vi "Experiment header-Save_Load STATS for Z-stack26_01_18.vi"(8 "error in (no error)":errorcluster, 10 "Function":enum16{"Write", "Read"}(ring), 11 "Experiment folder path":path) -> (0 "error out":errorcluster)   [LabVIEW 2017]
uses:
  Global Variables/General Globals.vi
  <vilib>/Utility/config.llb/Write Key (Double).vi
  <vilib>/Utility/config.llb/NI_LVConfig.lvlib
  <vilib>/Utility/config.llb/Read Key (Double).vi
panel:
  out "Z-stack duration (sec)":dbl
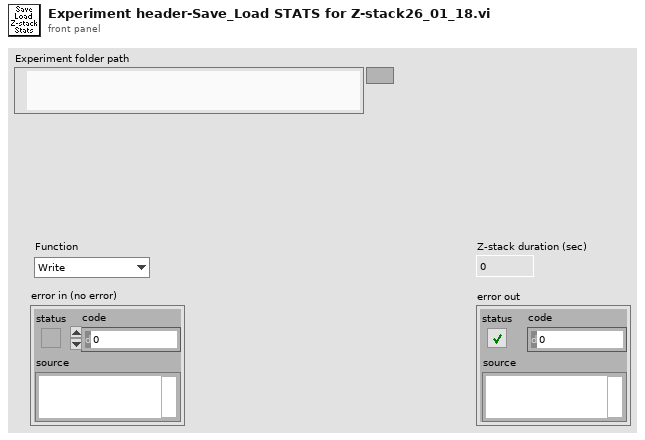
[diagram p1: front panel]
types:
  T1 = typedef "Fixed strings.ctl" = cluster{"ROI file name":string, "Normalised ROI file name":string, "Zplane Pockels values file name":string, "Functional data folder name":string, "Experiment Header file name":string, "Z-stack images folder name":string, "Groups setup rel. path":string, "Groups text file rel. path":string, "TDMS files folder name (F.img)":string, "TDMS files folder name (V.acq)":string, "TDMS files folder name (Pl.acq)":string, "Cycle rel times sequence file":string, "Dynamically called VIs folder name":string, "Time Series folder base name":string}
  T2 = typedef "NI_LVConfig.lvlib/Config Data RefNum.ctl" = refnum<k1>
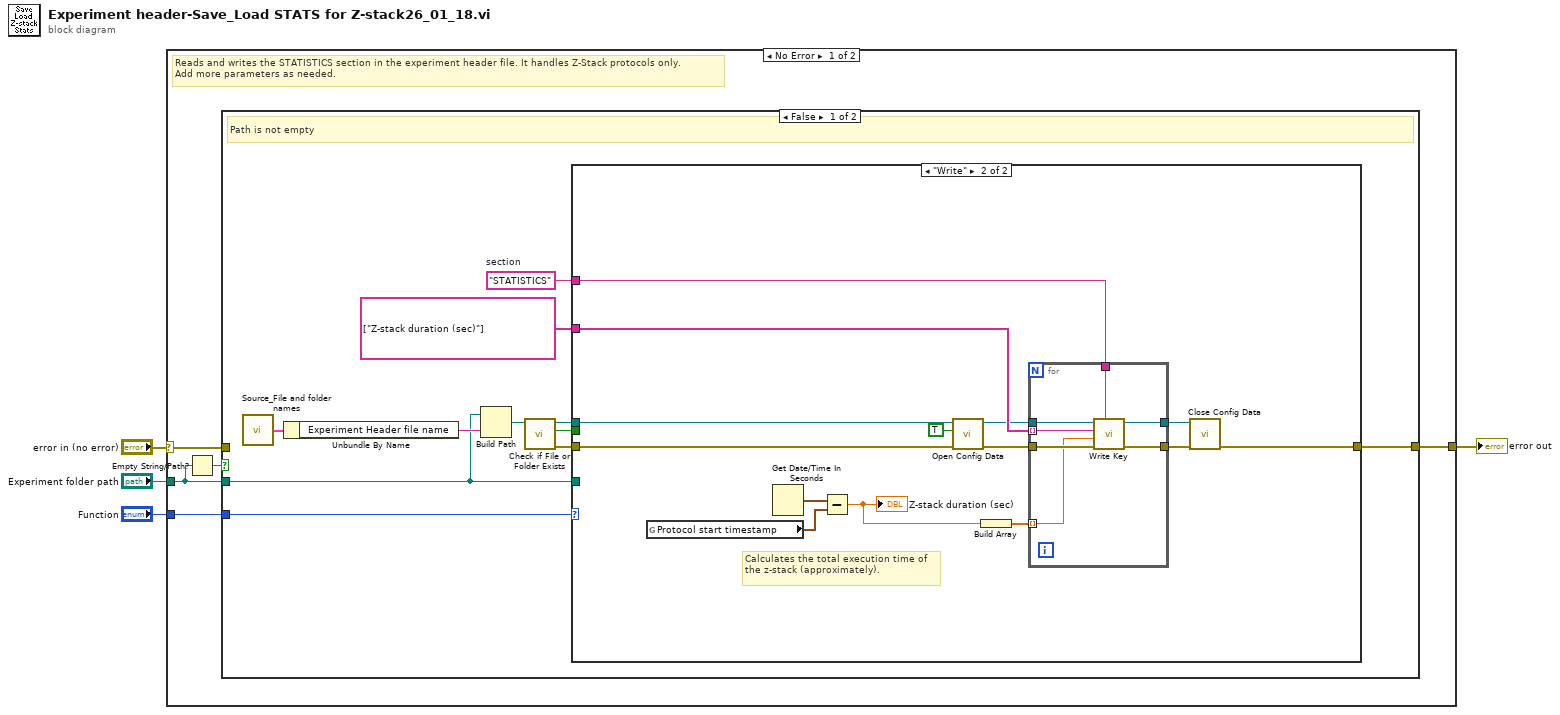
[diagram p0: block diagram]
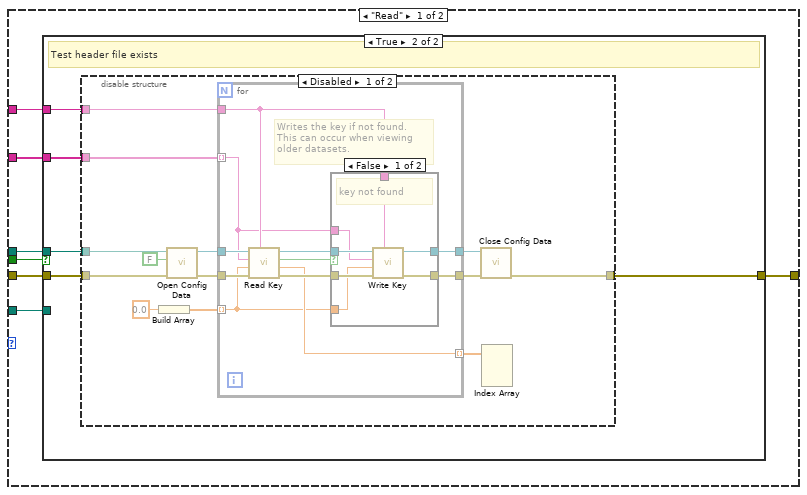
[diagram p2: hidden frame]
diagram:
  n1 = case shown="No Error" "error in (no error)" {
    selector: "error in (no error)" -> [w5 w89]
    tunnel: [w9 w89] -> w4
    tunnel: "Function" -> [w8 _]
    tunnel: "Experiment folder path" -> [w6 _]
    frame No Error {
      # "Reads and writes the STATISTICS section in the experiment header file. It handles Z-Stack protocols only.\nAdd more parameters as needed."
      n2 = Empty String/Path?(string/path=w6) -> (empty?=w7:bool)
      n3 = case shown="False" w7 {
        tunnel: [w10 w88] -> w9
        tunnel: w8 -> [w14 _]
        tunnel: w6 -> [w15 _]
        tunnel: w5 -> [_ w88]
        frame False {
          w16 = "STATISTICS"  # section
          # "Path is not empty"
          n4 = call "Source_File and folder names.vi"() -> ("Fixed strings"=w18:T1)  [unwired: 1 in]
          n5 = Unbundle By Name(w18) -> ("Experiment Header file name"=w19:string)
          n6 = Build Path(base path=w15, name or relative path=w19) -> (appended path=w17:path)
          n7 = call <vilib>:"Check if File or Folder Exists.vi"("path"=w17) -> ("error out"=w11:errorcluster, "file or folder exists?"=w13:bool, "dup path"=w12:path)  [unwired: 8 in]
          n8 = case shown="\"Write\"" w14 {
            tunnel: [w26 w72] -> w10
            tunnel: w11 -> [w27 w76]
            tunnel: w16 -> [w25 w80]
            tunnel: string[] ["Z-stack duration (sec)"] -> [w24 w79]
            tunnel: w15 -> [w23 _]
            tunnel: w13 -> [w21 _]
            tunnel: w12 -> [w22 w77]
            frame "Read" {
              n9 = case shown="True" w21 {
                tunnel: w27 -> [w28 w30]
                tunnel: [w28 w29] -> w26
                tunnel: w25 -> [_ w33]
                tunnel: w24 -> [_ w32]
                tunnel: w23 -> [_ _]
                tunnel: w22 -> [_ w31]
                frame False {
                  # "Test header file doesnot exist"
                }
                frame True {
                  # "Test header file exists"
                  n10 = disable-structure shown="Disabled" {
                    disable-tunnel: w33 -> [w46 _]
                    disable-tunnel: w32 -> [w45 _]
                    disable-tunnel: w31 -> [w43 _]
                    disable-tunnel: w30 -> [w40 _]
                    disable-tunnel: [w36 _] -> w29
                    frame Disabled {
                      n11 = Build Array(0.0 ("Number of acquired frames")) -> (w34:dbl[])
                      n12 = call <vilib>:"Open Config Data.vi"("error in (no error)"=w40, "create file if necessary (T)"=FALSE, "configuration file path"=w43) -> ("error out"=w39:errorcluster, "refnum"=w41:T2)  [unwired: 6 in, 1 out]
                      n13 = for {
                        tunnel: w41 -> [w57]
                        tunnel: w39 -> [w56]
                        tunnel: [w53] -> w38
                        tunnel: [w52] -> w37
                        tunnel: w46 -> [w51]
                        tunnel: [w49] -> w44 mode=indexing
                        tunnel: w34 -> [w47] mode=indexing
                        tunnel: w45 -> [w48] mode=indexing
                        # "Writes the key if not found.\nThis can occur when viewing older datasets."
                        n14 = call-poly <vilib>:"Read Key.vi"("section"=w51, "error in (no error)"=w56, "default value"=w47, "key"=w48, "refnum"=w57) -> ("error out"=w54:errorcluster, "value"=w49:dbl, "found?"=w50:bool, "refnum out"=w55:T2)  [unwired: 3 in]
                        n15 = case shown="False" w50 {
                          tunnel: w55 -> [w64 w66]
                          tunnel: w54 -> [w63 w65]
                          tunnel: [w62 w66] -> w53
                          tunnel: [w61 w65] -> w52
                          tunnel: w51 -> [w60 _]
                          tunnel: w48 -> [w59 _]
                          tunnel: w47 -> [w58 _]
                          frame False {
                            # "key not found"
                            n16 = call-poly <vilib>:"Write Key.vi"("section"=w60, "error in (no error)"=w63, "value"=w58, "key"=w59, "refnum"=w64) -> ("error out"=w61:errorcluster, "refnum out"=w62:T2)  [unwired: 4 in, 1 out]
                          }
                          frame True {
                            # "found"
                          }
                        }
                      }
                      n17 = call <vilib>:"Close Config Data.vi"("error in (no error)"=w37, "refnum"=w38) -> ("error out"=w36:errorcluster)  [unwired: 8 in, 1 out]
                      n18 = Index Array(array=w44) -> ()  [unwired: 3 in, 3 out]
                    }
                    frame Enabled {
                    }
                  }
                }
              }
            }
            frame "Write" {
              # "Calculates the total execution time of the z-stack (approximately)."
              n19 = global read "General Globals.vi" "Protocol start timestamp"() -> (w69:timestamp)
              n20 = Get Date/Time In Seconds() -> (seconds since 1Jan1904=w68:timestamp)
              n21 = Subtract(x=w68, y=w69) -> (x-y=w67:dbl)
              "Z-stack duration (sec)" <- w67
              n22 = call <vilib>:"Open Config Data.vi"("error in (no error)"=w76, "create file if necessary (T)"=TRUE, "configuration file path"=w77) -> ("error out"=w75:errorcluster, "refnum"=w78:T2)  [unwired: 6 in, 1 out]
              n23 = Build Array(w67) -> (w70:dbl[])
              n24 = for {
                tunnel: w78 -> [w87]
                tunnel: w75 -> [w86]
                tunnel: w79 -> [w85] mode=indexing
                tunnel: w80 -> [w84]
                tunnel: [w83] -> w71
                tunnel: [w82] -> w73
                tunnel: w70 -> [w81] mode=indexing
                n25 = call-poly <vilib>:"Write Key.vi"("section"=w84, "error in (no error)"=w86, "value"=w81, "key"=w85, "refnum"=w87) -> ("error out"=w83:errorcluster, "refnum out"=w82:T2)  [unwired: 4 in, 1 out]
              }
              n26 = call <vilib>:"Close Config Data.vi"("error in (no error)"=w71, "refnum"=w73) -> ("error out"=w72:errorcluster)  [unwired: 8 in, 1 out]
            }
          }
        }
        frame True {
          # "Empty path"
        }
      }
    }
    frame Error {
    }
  }
  "error out" <- w4
